vi "Run.vi"(8 "error in (no error)":errorcluster, 11 "SB App in":refnum<class "SB App.lvclass">) -> (0 "error out":errorcluster, 3 "SB App out":refnum<class "SB App.lvclass">)   [LabVIEW 2020, in "SB App.lvlib" / "SB App.lvclass"]
uses:
  SB App.lvclass
  SB App.lvclass/SB App.ctl
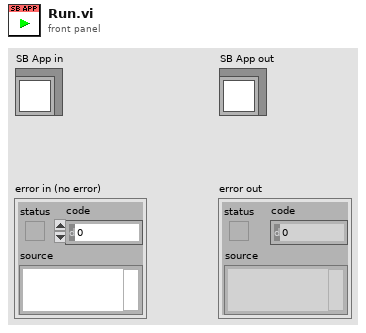
[diagram p1: front panel]
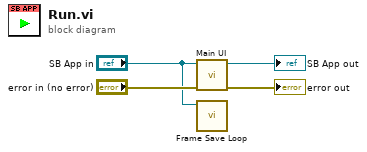
[diagram p0: block diagram]
diagram:
  n1 = call "Main UI.vi"("error in (no error)"="error in (no error)", "SB App in"="SB App in") -> ("error out"=→"error out":errorcluster, "SB App out"=→"SB App out":refnum<class "SB App.lvclass">)  [unwired: 8 in]
  n2 = call "Frame Save Loop.vi"("SB App in"="SB App in") -> ()  [unwired: 10 in, 1 out]
